vi "LT_init_sn.vi"(6 "SN":string, 7 "do_reset":bool=TRUE, 8 "error in":errorcluster, 9 "Converter Type\n(180: Turbovac 350/450 i)":T3=187 items=["Turbovac 350/450 i"=180, "Turbovac 350/450 i with optional interface"=181, "Turbovac 350/450 iX"=182, "Turbovac 90/250 i"=190, "Turbovac 90/250 with optional interface"=191, "Turbovac 90/250 iX"=192, "TURBOVAC 850/950 i"=195, "TURBOVAC 850/950 i with optional interface"=196, "TURBOVAC 850/950 iX"=197, "TURBOVAC 1300 i"=185, "TURBOVAC 1300 i with optional interface"=186, "TURBOVAC 1300 iX"=187], 10 "Converter address (0)":u8, 11 "VISA in":refnum<visa-resource-name>="COM43") -> (0 "error out":errorcluster, 2 "dev_param_out":T1={"Length of data block"=14, "Converter address"=0, "Converter type"=180, "PZD1"=0, "PZD2"=0} {"Converter type" items=["Turbovac 350/450 i"=180, "Turbovac 350/450 i with optional interface"=181, "Turbovac 350/450 iX"=182, "Turbovac  90/250 i"=190, "Turbovac  90/250 with optional interface"=191, "Turbovac  90/250 iX"=192, "Turbovac  850/950 i"=195, "Turbovac  850/950 i with optional interface"=196, "Turbovac  850/950 iX"=197, "Turbovac 1350/1450 i"=185, "Turbovac 1350/1450 i with optional interface"=186, "Turbovac 1350/1450 iX"=187]; "Length of data block" items=["14"=14, "22"=22]}, 3 "VISA out":refnum<visa-resource-name>, 4 "status":bool)   [LabVIEW 2019]
doc: "Example VI to demonstrate the use of the Oerlikon Leybold TMP driver."
uses:
  <instrlib>/Leybold TURBOVAC/Public/Ctl/Converter Type Control.ctl
  <instrlib>/Leybold TURBOVAC/Public/Ctl/Device Parameters Indicator.ctl
  <instrlib>/Leybold TURBOVAC/Public/Ctl/Converter Type Indicator.ctl
  <vilib>/Utility/error.llb/Error Cluster From Error Code.vi
  <vilib>/ErrorRing/Error Ring.xnode
  <instrlib>/Leybold TURBOVAC/Leybold TURBOVAC.lvlib
panel:
  # "The converter address and type don't matter\nsince we use the remote drive unit (iR) via USB."
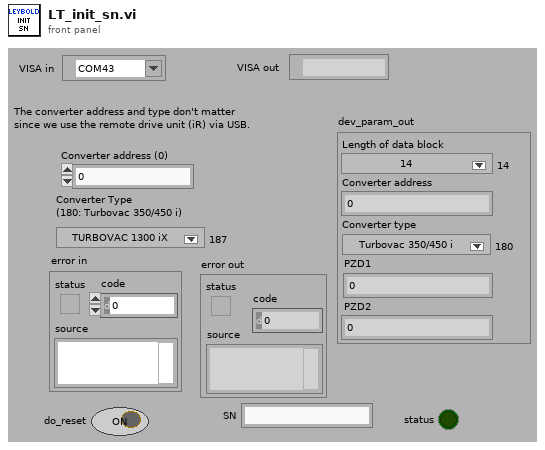
[diagram p1: front panel]
types:
  T1 = typedef "Leybold TURBOVAC.lvlib/Device Parameters Indicator.ctl" = cluster{"Length of data block":u8, "Converter address":u8, "Converter type":T2, "PZD1":u16, "PZD2":u16}
  T2 = typedef "Leybold TURBOVAC.lvlib/Converter Type Indicator.ctl" = u16
  T3 = typedef "Leybold TURBOVAC.lvlib/Converter Type Control.ctl" = u16
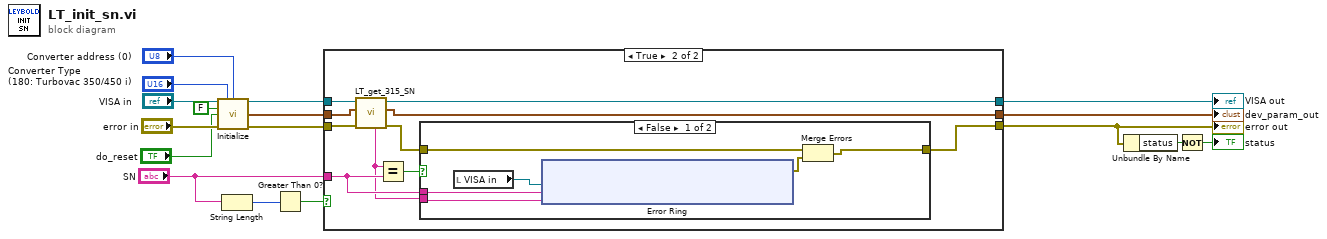
[diagram p0: block diagram]
diagram:
  n1 = call <instrlib>:"Initialize.vi"("VISA resource name"="VISA in", "Converter Type\n(180: Turbovac 350/450 i)"="Converter Type\n(180: Turbovac 350/450 i)", "Converter address (0)"="Converter address (0)", "ID Query? (T: Yes)"=FALSE, "Reset? (T: Yes)"="do_reset", "error in (no error)"="error in") -> ("VISA resource name out"=w11:refnum<visa-resource-name>, "Device parameters out"=w7:T1, "error out"=w9:errorcluster)  [unwired: 7 in]
  n2 = String Length(string="SN") -> (length=w6:i32)
  n3 = Greater Than 0?(x=w6) -> (x > 0?=w5:bool)
  n4 = case shown="True" w5 {
    tunnel: w11 -> [w20 w30]
    tunnel: [w20 w29] -> w10
    tunnel: w9 -> [w18 w28]
    tunnel: [w18 w23] -> w3
    tunnel: [w19 w27] -> w8
    tunnel: w7 -> [w19 w26]
    tunnel: "SN" -> [_ w22]
    frame False {
    }
    frame True {
      n5 = call "LT_get_315_SN.vi"("error in"=w28, "dev_param_in"=w26, "VISA in"=w30) -> ("error out"=w24:errorcluster, "dev_param_out"=w27:T1, "VISA out"=w29:refnum<visa-resource-name>, "SN_converter"=w21:string)  [unwired: 5 in]
      n6 = Equal?(x=w21, y=w22) -> (x = y?=w25:bool)
      n7 = case shown="False" w25 {
        tunnel: w24 -> [w36 w46]
        tunnel: [w34 w46] -> w23
        tunnel: w22 -> [w32 _]
        tunnel: w21 -> [w31 _]
        frame False {
          n8 = local read "VISA in"() -> (w33:refnum<visa-resource-name>)
          n9 = xnode "Error Ring"("parameter 0"=w33, "parameter 1"=w32, "parameter 2"=w31) -> ("error out"=w35:errorcluster)
          n10 = Merge Errors(w36, w35) -> (w34:errorcluster)
        }
        frame True {
        }
      }
    }
  }
  "VISA out" <- w10
  "dev_param_out" <- w8
  "error out" <- w3
  n11 = Unbundle By Name(w3) -> ("status"=w2:bool)
  n12 = Not(x=w2) -> (.not. x?=→"status":bool)
